vi "FIND TURE FOR AUTO.vi"(9 "CYCLE START":bool) -> (3 "Boolean":bool)   [LabVIEW 2017]
uses:
  <userlib>/_OpenG.lib/comparison/comparison.llb/Boolean Changed__ogtk.vi
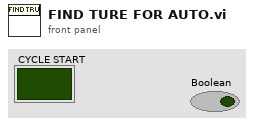
[diagram p1: front panel]
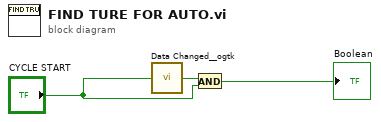
[diagram p0: block diagram]
diagram:
  n1 = call-poly <userlib>:"Data Changed__ogtk.vi"("Boolean"="CYCLE START") -> ("Changed"=w2:bool)
  n2 = And(x=w2, y="CYCLE START") -> (x .and. y?=→"Boolean":bool)
